vi "Channel Get Mapping.vi"(8 "error in (no error)":errorcluster, 11 "Item Ref in":T1 format="%.0x") -> (0 "error out":errorcluster, 2 "Mapping":T2 {"VS Reference" format="%.0x"}, 3 "Item Ref out":T1 format="%.0x")   [LabVIEW 2021, in "Modbus Master System Explorer.lvlib"]
uses:
  Modbus Master System Explorer.lvlib
  <vilib>/NI VeriStand/Custom Device API/Custom Device Item Ref.ctl
  Shared/Controls/Data Model/Mapping.ctl
  Shared/Controls/Data Model/DataType.ctl
  Shared/Modbus Master Shared.lvlib
  <vilib>/NI VeriStand/Custom Device API/Custom Device API.lvlib
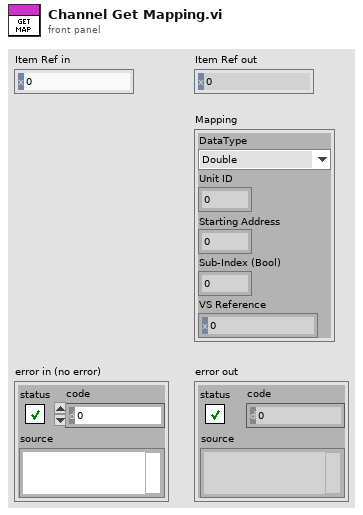
[diagram p1: front panel]
types:
  T1 = typedef "Custom Device API.lvlib/Custom Device Item Ref.ctl" = u64
  T2 = typedef "Modbus Master Shared.lvlib/Mapping.ctl" = cluster{"DataType":T3, "Unit ID":u8, "Starting Address":u16, "Sub-Index (Bool)":u16, "VS Reference":T1}
  T3 = typedef "Modbus Master Shared.lvlib/DataType.ctl" = enum16{"Double", "Single", "I64", "I32", "I16", "I8", "U64", "U32", "U16", "U8", "Boolean"}
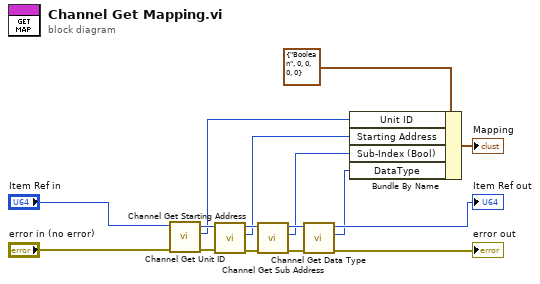
[diagram p0: block diagram]
diagram:
  n1 = call "Channel Get Unit ID.vi"("error in (no error)"="error in (no error)", "Item Ref in"="Item Ref in") -> ("error out"=w4:errorcluster, "Value"=w1:u8, "Item Ref out"=w5:T1)  [unwired: 7 in]
  n2 = call "Channel Get Starting Address.vi"("error in (no error)"=w4, "Item Ref in"=w5) -> ("error out"=w13:errorcluster, "Value"=w8:u16, "Item Ref out"=w14:T1)  [unwired: 7 in]
  n3 = call "Channel Get Sub Address.vi"("error in (no error)"=w13, "Item Ref in"=w14) -> ("error out"=w11:errorcluster, "Value"=w7:u16, "Item Ref out"=w12:T1)  [unwired: 7 in]
  n4 = call "Channel Get Data Type.vi"("error in (no error)"=w11, "Item Ref in"=w12) -> ("error out"=→"error out":errorcluster, "Data Type"=w6:T3, "Item Ref out"=→"Item Ref out":T1)  [unwired: 7 in]
  n5 = Bundle By Name(cluster=T2 {"DataType"=enum."Boolean", "Unit ID"=0, "Starting Address"=0, "Sub-Index (Bool)"=0, "VS Reference"=0} ("Mapping"), "Unit ID"=w1, "Starting Address"=w8, "Sub-Index (Bool)"=w7, "DataType"=w6) -> (→"Mapping":T2)
